vi "Write Prepend Result Name.vi"(8 "error in (no error)":errorcluster, 10 "Prepend Result Name":bool, 11 "SeqAuto IEvaluation in":refnum<class "SeqAuto IEvaluation.lvclass">) -> (0 "error out":errorcluster, 3 "SeqAuto IEvaluation out":refnum<class "SeqAuto IEvaluation.lvclass">)   [LabVIEW 2018, in "IEvaluation.lvlib" / "SeqAuto IEvaluation.lvclass"]
uses:
  SeqAuto IEvaluation.lvclass
  SeqAuto IEvaluation.lvclass/SeqAuto IEvaluation.ctl
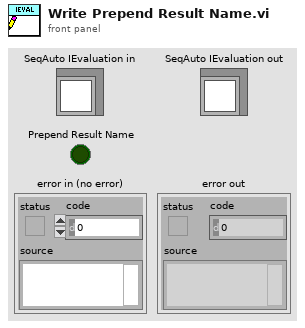
[diagram p1: front panel]
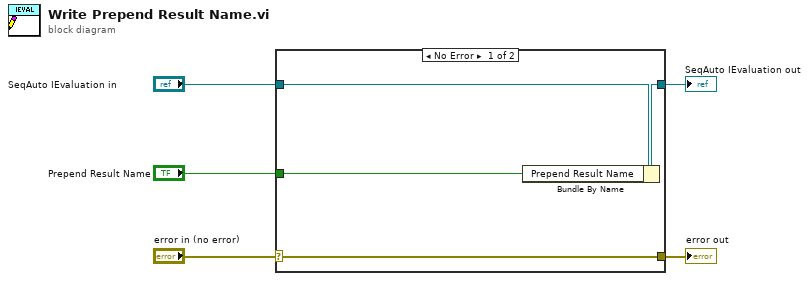
[diagram p0: block diagram]
diagram:
  n1 = case shown="No Error" "error in (no error)" {
    selector: "error in (no error)" -> [w9 w10]
    tunnel: [w9 w10] -> w4
    tunnel: [w7 w11] -> w2
    tunnel: "SeqAuto IEvaluation in" -> [w8 w11]
    tunnel: "Prepend Result Name" -> [w6 _]
    frame No Error {
      n2 = Bundle By Name(cluster=w8, "Prepend Result Name"=w6) -> (w7:refnum<class "SeqAuto IEvaluation.lvclass">)
    }
    frame Error {
    }
  }
  "error out" <- w4
  "SeqAuto IEvaluation out" <- w2
